vi "Configure Waveform Characteristics.vi"(5 "Waveform Count (1)":i32=1, 6 "Waveform Last Termination (False: Off)":bool, 7 "Waveform Shape (0: None)":i32(ring) items=["None", "Constant Dwell", "Exponential", "Pulse", "Ramp", "Sine Wave", "Staircase", "Step", "Trapezoid", "Sequence", "User Defined"], 8 "error in (no error)":errorcluster {"code" format="%.0x"}, 9 "Waveform Type (1: Voltage)":i32(ring)=1 items=["Voltage"=1, "Current"=0], 10 "Channel Name (1)":string="1", 11 "VISA resource name":refnum<visa-resource-name>) -> (0 "error out":errorcluster {"code" format="%.0x"}, 3 "VISA resource name out":refnum<visa-resource-name>)   [LabVIEW 2016, in "Agilent N6700 Series.lvlib"]
doc: "Sets the waveform type, shape, count and the output value when the waveform terminates. \n\n<b>Note:</b>\nThis VI only applies to the N6705B and N6705C DC Power Analyzer."
uses:
  <instrlib>/Agilent N6700 Series/Agilent N6700 Series.lvlib
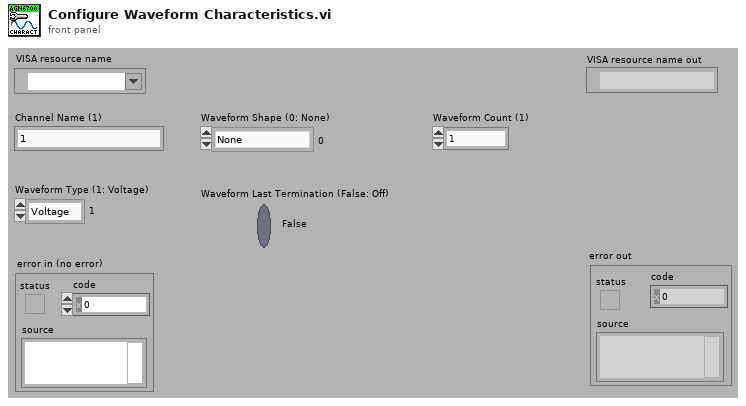
[diagram p1: front panel]
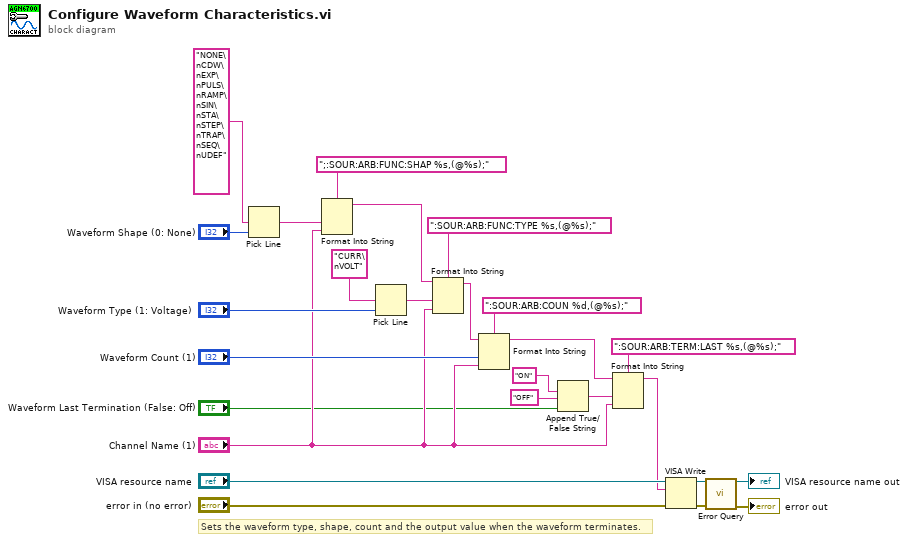
[diagram p0: block diagram]
diagram:
  # "Sets the waveform type, shape, count and the output value when the waveform terminates."
  n1 = Pick Line(multi-line string="NONE\nCDW\nEXP\nPULS\nRAMP\nSIN\nSTA\nSTEP\nTRAP\nSEQ\nUDEF" ("string (\"\")"), line index="Waveform Shape (0: None)") -> (output string=w19:string)  [unwired: 1 in]
  n2 = Format Into String(format string=";:SOUR:ARB:FUNC:SHAP %s,(@%s);", w19, "Channel Name (1)") -> (resulting string=w12:string)  [unwired: 2 in, 1 out]
  n3 = Pick Line(multi-line string="CURR\nVOLT" ("string (\"\")"), line index="Waveform Type (1: Voltage)") -> (output string=w16:string)  [unwired: 1 in]
  n4 = Format Into String(format string=":SOUR:ARB:FUNC:TYPE %s,(@%s);", initial string=w12, w16, "Channel Name (1)") -> (resulting string=w5:string)  [unwired: 1 in, 1 out]
  n5 = Format Into String(format string=":SOUR:ARB:COUN %d,(@%s);", initial string=w5, "Waveform Count (1)", "Channel Name (1)") -> (resulting string=w4:string)  [unwired: 1 in, 1 out]
  n6 = Append True/False String(1:"Waveform Last Termination (False: Off)", 2:"OFF", 3:"ON") -> (0:w11:string)  [unwired: 1 in]
  n7 = Format Into String(format string=":SOUR:ARB:TERM:LAST %s,(@%s);", initial string=w4, w11, "Channel Name (1)") -> (resulting string=w3:string)  [unwired: 1 in, 1 out]
  n8 = VISA Write(VISA resource name="VISA resource name", write buffer=w3, error in (no error)="error in (no error)") -> (VISA resource name out=w22:refnum<visa-resource-name>, error out=w21:errorcluster)  [unwired: 1 out]
  n9 = call <instrlib>:"Error Query.vi"("VISA resource name"=w22, "error in (no error)"=w21) -> ("VISA resource name out"=→"VISA resource name out":refnum<visa-resource-name>, "error out"=→"error out":errorcluster)  [unwired: 10 in, 2 out]
